vi "verify executabiity of line.vi"(9 "Freq multiplication factor":i32=9 min=9 max=108 step=3, 10 "Instr status":T2, 11 "Script cluster":T1={"Start"=0.0, "Start Caption"="Start [T]", "End"=0.0, "End Caption"="End [T]", "Sweep"=0.0, "Sweep caption"="Rate [mT/s]", "Constant"=0.0, "Constant caption"="Freq [GHz]", "Mod_F [kHz]"=0.0, "Mod_A [G]"=0.0, "Tau [ms]"=0.0, "Angle [°]"=0.0, "Tmp [K]"=50.0, "Wait [min]"=0.0, "Carousel"=-1, "Comment"="", "Auto-mod"=TRUE, "Execute"=FALSE} {"Carousel" items=["0", "1", "2", "3", "4", "5", "6"]; "Angle [°]" min=0.0 max=350.0; "Tau [ms]" min=0.0 max=100.0; "Wait [min]" min=0.0 max=350.0; "Tmp [K]" min=0.0 max=3000.0; "Mod_A [G]" min=0.1 max=150.0; "Mod_F [kHz]" min=0.1 max=150.0}) -> (2 "Response":string, 3 "is executable":bool)   [LabVIEW 2024]
doc: "Checks (VTI and multipiers) if line of script is executable."
uses:
  Datatypes/Mudules status.ctl
  Datatypes/script polymorh line.ctl
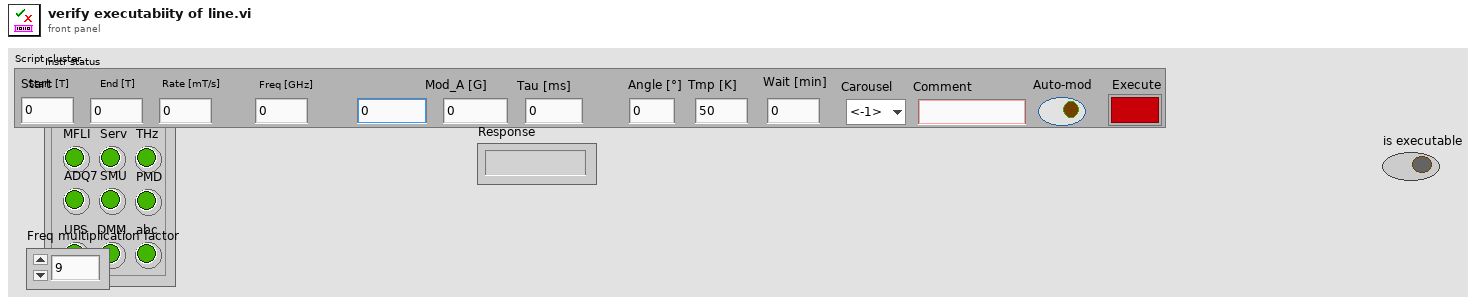
[diagram p1: front panel]
types:
  T1 = typedef "script polymorh line.ctl" = cluster{"Start":dbl, "Start Caption":string, "End":dbl, "End Caption":string, "Sweep":dbl, "Sweep caption":string, "Constant":dbl, "Constant caption":string, "Mod_F [kHz]":dbl, "Mod_A [G]":dbl, "Tau [ms]":dbl, "Angle [°]":dbl, "Tmp [K]":dbl, "Wait [min]":dbl, "Carousel":i8, "Comment":string, "Auto-mod":bool, "Execute":bool}
  T2 = typedef "Mudules status.ctl" = cluster{"Mag":bool, "Rot":bool, "VTI":bool, "MFLI":bool, "Serv":bool, "THz":bool, "ADQ7":bool, "SMU":bool, "PMD":bool, "UPS":bool, "DMM":bool, "abc":bool}
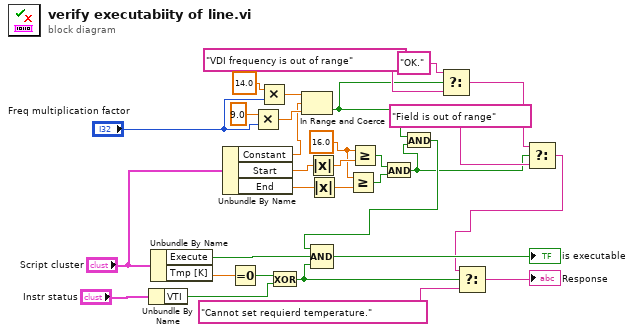
[diagram p0: block diagram]
diagram:
  w7 = 16.0 ("y")
  n1 = Unbundle By Name("Instr status") -> ("VTI"=w28:bool)
  n2 = Unbundle By Name("Script cluster") -> ("Execute"=w26:bool, "Tmp [K]"=w30:dbl)
  n3 = Unbundle By Name("Script cluster") -> ("Constant"=w11:dbl, "Start"=w8:dbl, "End"=w9:dbl)
  n4 = Equal To 0?(x=w30) -> (x = 0?=w29:bool)
  n5 = Multiply(x=9.0, y="Freq multiplication factor") -> (x*y=w12:dbl)
  n6 = Multiply(x=14.0, y="Freq multiplication factor") -> (x*y=w18:dbl)
  n7 = Exclusive Or(1:w28, 2:w29) -> (0:w25:bool)
  n8 = In Range and Coerce(upper limit=w18, x=w11, lower limit=w12) -> (In Range?=w1:bool)  [unwired: 1 out]
  n9 = Absolute Value(x=w8) -> (abs(x)=w10:dbl)
  n10 = Absolute Value(x=w9) -> (abs(x)=w6:dbl)
  n11 = Greater Or Equal?(x=w7, y=w6) -> (x >= y?=w4:bool)
  n12 = Greater Or Equal?(x=w7, y=w10) -> (x >= y?=w5:bool)
  n13 = And(x=w5, y=w4) -> (x .and. y?=w2:bool)
  n14 = And(x=w1, y=w2) -> (x .and. y?=w22:bool)
  n15 = Compound Arithmetic op=AND(w22, w26, w25) -> (→"is executable":bool)
  n16 = Select(t="OK.", s=w1, f="VDI frequency is out of range") -> (s? t:f=w13:string)
  n17 = Select(t=w13, s=w2, f="Field is out of range") -> (s? t:f=w21:string)
  n18 = Select(t=w21, s=w25, f="Cannot set requierd temperature.") -> (s? t:f=→"Response":string)
